vi "Prepend Length.vi"(8 "error in (no error)":errorcluster, 10 "JSON Response String in":string) -> (0 "error out":errorcluster, 2 "JSON Response String out":string)   [LabVIEW 2020, in "RPC.lvlib"]
uses:
  RPC.lvlib
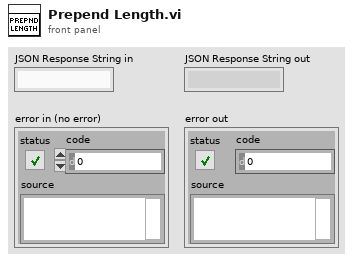
[diagram p1: front panel]
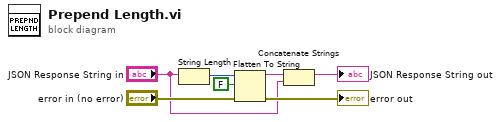
[diagram p0: block diagram]
diagram:
  n1 = String Length(string="JSON Response String in") -> (length=w7:i32)
  n2 = Flatten To String(anything=w7, prepend array or string size? (T)=FALSE, error in (no error)="error in (no error)") -> (data string=w3:string, error out=→"error out":errorcluster)  [unwired: 1 in, 1 out]
  n3 = Concatenate Strings(w3, "JSON Response String in") -> (→"JSON Response String out":string)
